vi "MSP6715-OnOff.vi"(8 "error in":errorcluster caption="错误输入（无错误）", 10 "On_Off":bool, 11 "MyIndex":u8) -> (0 "error out":errorcluster)   [LabVIEW 2015, in "MSP6715.lvlib"]
uses:
  MSP6715.lvlib
  <vilib>/Instr/_visa.llb/VISA Configure Serial Port (Instr).vi
panel:
  out "返回值":u8[](array[numeric])
  in  "等待时间(毫秒)":u32=100
  out "VISA":refnum<visa-resource-name>
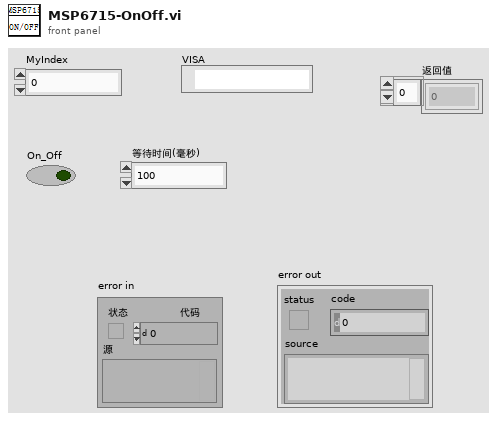
[diagram p1: front panel]
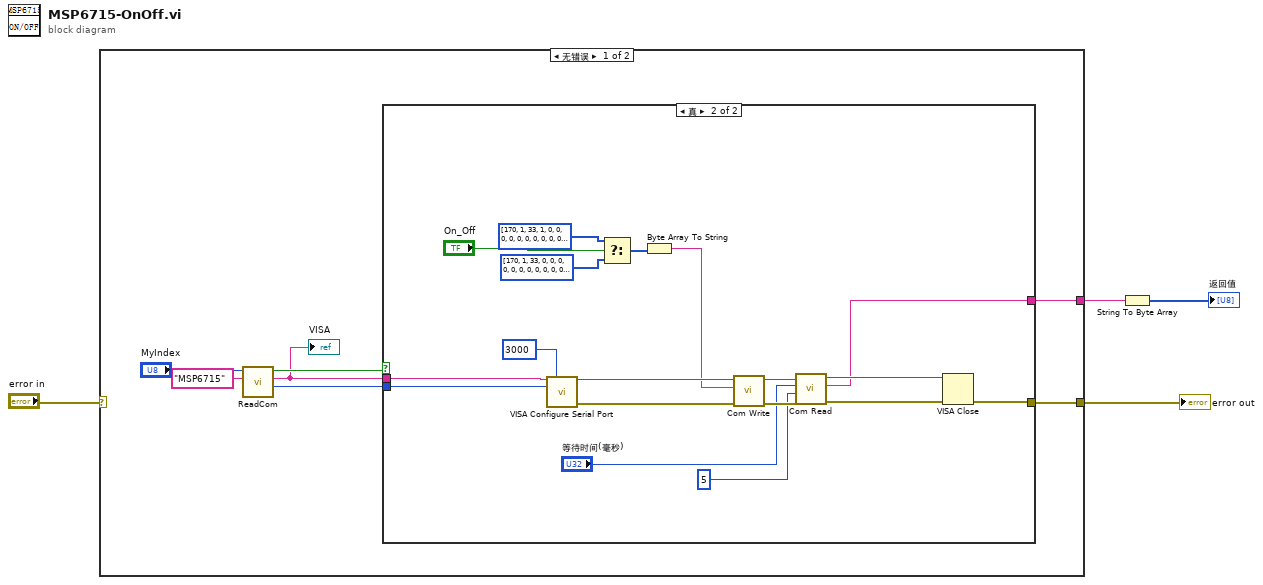
[diagram p0: block diagram]
diagram:
  n1 = case shown="无错误" "error in" {
    selector: "error in" -> [_ w30]
    tunnel: [w11 w30] -> w4
    tunnel: [w5 _] -> w2
    frame No Error {
      n2 = call "ReadCom.vi"("仪器名称"="MSP6715", "MyIndex"="MyIndex") -> ("Baudrate"=w6:i32, "COM"=w7:string, "OK?"=w8:bool)  [unwired: 7 in]
      "VISA" <- w7
      n3 = case shown="真" w8 {
        tunnel: [_ w29] -> w11
        tunnel: w7 -> [_ w28]
        tunnel: w6 -> [_ w27]
        tunnel: [_ w19] -> w5
        frame False {
        }
        frame True {
          n4 = call-poly "VISA Configure Serial Port"("VISA resource name"=w28, "timeout (10sec)"=u32 3000, "baud rate (9600)"=w27) -> ("VISA resource name out"=w25:refnum<visa-resource-name>, "error out"=w24:errorcluster)  [unwired: 11 in]
          n5 = Select(t=u32[] [170, 1, 33, 1, 0, 0, 0, 0, 0, 0, 0, 0, 0, 0, 0, 0, 0, 0, 0, 0, 0, 0, 0, 0, 0, 205] ("Hex指令"), s="On_Off", f=u32[] [170, 1, 33, 0, 0, 0, 0, 0, 0, 0, 0, 0, 0, 0, 0, 0, 0, 0, 0, 0, 0, 0, 0, 0, 0, 204] ("Hex指令")) -> (s? t:f=w16:u32[])
          n6 = Byte Array To String(unsigned byte array=w16) -> (string=w12:string)
          n7 = call "Com Write.vi"("错误输入（无错误）"=w24, "Wbuff"=w12, "VISA In"=w25) -> ("错误输出"=w22:errorcluster, "VISA Out"=w23:refnum<visa-resource-name>)  [unwired: 7 in]
          n8 = call "Com Read.vi"("错误输入（无错误）"=w22, "num"=u32 5, "超时"="等待时间(毫秒)", "VISA In"=w23) -> ("错误输出"=w21:errorcluster, "buff"=w19:string, "VISA Out"=w20:refnum<visa-resource-name>)  [unwired: 5 in]
          n9 = VISA Close(VISA resource name=w20, error in (no error)=w21) -> (error out=w29:errorcluster)
        }
      }
    }
    frame Error {
    }
  }
  "error out" <- w4
  n10 = String To Byte Array(string=w2) -> (unsigned byte array=→"返回值":u8[])
